vi "Set Velocity.vi"(0 "Process Variable(x)":dbl, 5 "Current TIme":u32, 7 "Current Power":dbl, 9 "Setpoint(end)":dbl, 11 "Total Distance":dbl format="%#_13g", 12 "Last Time Input":u32) -> (4 "Coerced Motor power":dbl format="%#_13g", 6 "End Loop?":bool=TRUE, 8 "Non-Coerced Motor Power":dbl, 10 "Last Time Output":u32)   [LabVIEW 2016]
panel:
  in  "Tick range":dbl=300.0 format="%#_13g"
  in  "Power Constant (power/ms^2) constant":dbl=0.0002 format="%#_13g"
  in  "Robot Barely Moving Power":dbl=0.3 format="%#_13g"
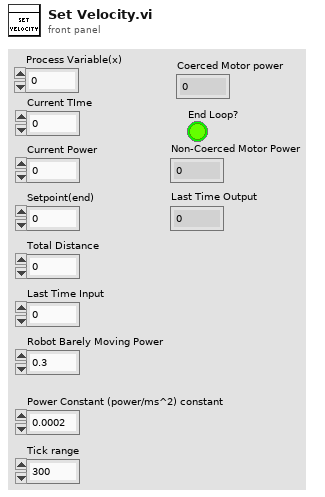
[diagram p1: front panel]
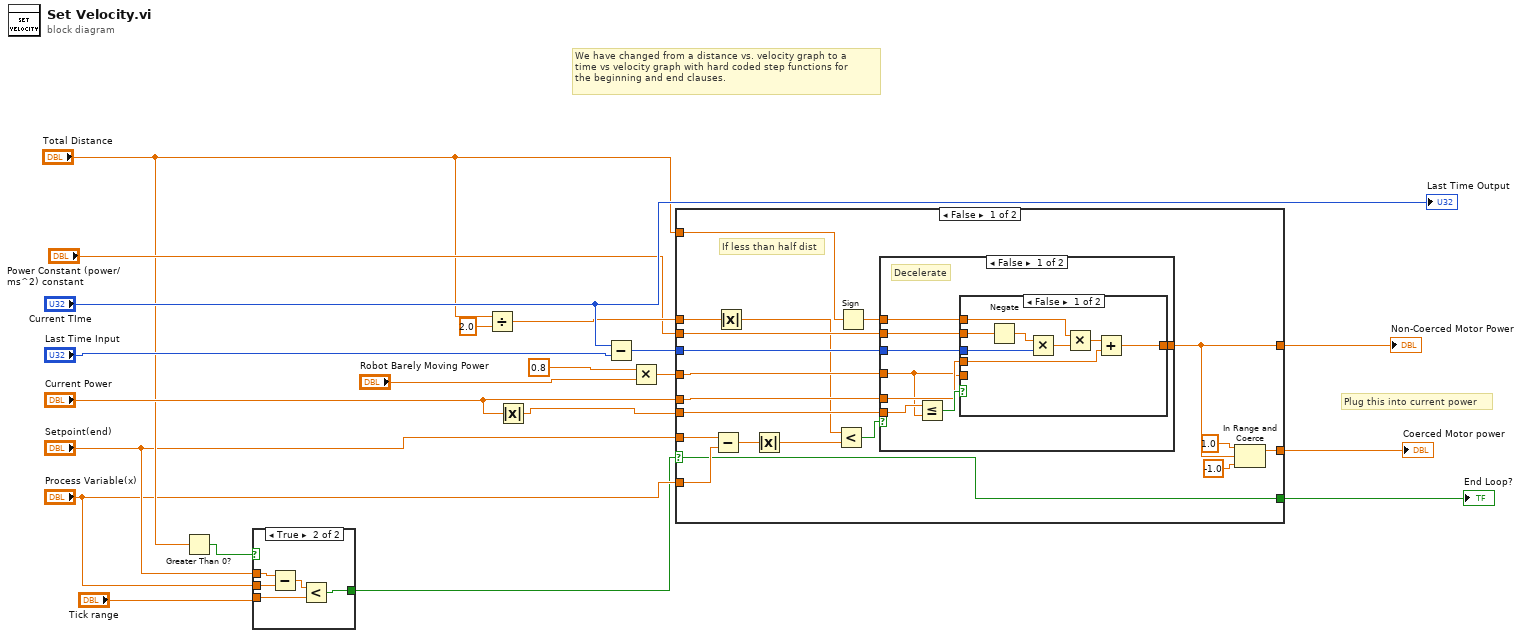
[diagram p0: block diagram]
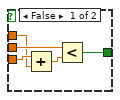
[diagram p2: hidden frame]
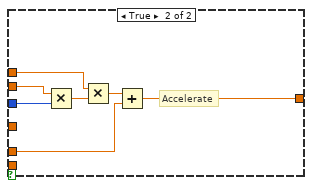
[diagram p4: hidden frame]
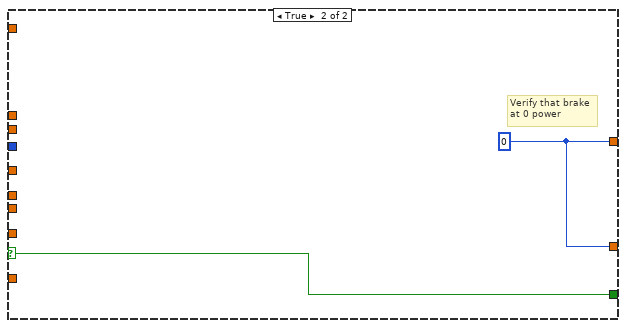
[diagram p5: hidden frame]
diagram:
  # "Plug this into current power"
  # "We have changed from a distance vs. velocity graph to a\ntime vs velocity graph with hard coded step functions for \nthe beginning and end clauses."
  n1 = Greater Than 0?(x="Total Distance") -> (x > 0?=w7:bool)
  n2 = case shown="True" w7 {
    tunnel: "Tick range" -> [w23 w30]
    tunnel: "Setpoint(end)" -> [w22 w29]
    tunnel: "Process Variable(x)" -> [w25 w28]
    tunnel: [w21 w26] -> w2
    frame False {
      n3 = Add(x=w23, y=w22) -> (x+y=w24:dbl)
      n4 = Less?(x=w25, y=w24) -> (x < y?=w21:bool)
    }
    frame True {
      n5 = Subtract(x=w29, y=w28) -> (x-y=w27:dbl)
      n6 = Less?(x=w27, y=w30) -> (x < y?=w26:bool)
    }
  }
  n7 = Divide(x="Total Distance", y=2.0) -> (x/y=w10:dbl)
  n8 = Absolute Value(x="Current Power") -> (abs(x)=w9:dbl)
  n9 = Subtract(x="Current TIme", y="Last Time Input") -> (x-y=w15:u32)
  n10 = Multiply(x=0.8, y="Robot Barely Moving Power") -> (x*y=w17:dbl)
  n11 = case shown="False" w2 {
    selector: w2 -> [w43 w75]
    tunnel: "Setpoint(end)" -> [w49 _]
    tunnel: "Process Variable(x)" -> [w48 _]
    tunnel: [w46 w74] -> w20
    tunnel: [w43 w75] -> w19
    tunnel: "Total Distance" -> [w41 _]
    tunnel: w10 -> [w40 _]
    tunnel: w17 -> [w36 _]
    tunnel: w15 -> [w39 _]
    tunnel: "Current Power" -> [w33 _]
    tunnel: w9 -> [w37 _]
    tunnel: "Power Constant (power/ms^2) constant" -> [w35 _]
    tunnel: [w32 w74] -> w1
    frame False {
      # "If less than half dist"
      n12 = Subtract(x=w49, y=w48) -> (x-y=w47:dbl)
      n13 = Absolute Value(x=w40) -> (abs(x)=w31:dbl)
      n14 = Absolute Value(x=w47) -> (abs(x)=w42:dbl)
      n15 = Less?(x=w31, y=w42) -> (x < y?=w38:bool)
      n16 = Sign(1:w41) -> (0:w34:dbl)
      n17 = case shown="False" w38 {
        tunnel: w39 -> [w53 w73]
        tunnel: [w55 w67] -> w32
        tunnel: w36 -> [w50 _]
        tunnel: w37 -> [w57 _]
        tunnel: w35 -> [w54 w71]
        tunnel: w34 -> [w52 w70]
        tunnel: w33 -> [w51 w68]
        frame False {
          # "Decelerate"
          n18 = Less Or Equal?(x=w57, y=w50) -> (x <= y?=w56:bool)
          n19 = case shown="False" w56 {
            tunnel: [w58 w66] -> w55
            tunnel: w50 -> [_ w66]
            tunnel: w54 -> [w64 _]
            tunnel: w53 -> [w63 _]
            tunnel: w52 -> [w61 _]
            tunnel: w51 -> [w59 _]
            frame False {
              n20 = Negate(x=w64) -> (-x=w65:dbl)
              n21 = Multiply(x=w65, y=w63) -> (x*y=w62:dbl)
              n22 = Multiply(x=w61, y=w62) -> (x*y=w60:dbl)
              n23 = Add(x=w60, y=w59) -> (x+y=w58:dbl)
            }
            frame True {
              # "Sets to barely moving power"
            }
          }
        }
        frame True {
          # "Accelerate"
          n24 = Multiply(x=w71, y=w73) -> (x*y=w72:dbl)
          n25 = Multiply(x=w70, y=w72) -> (x*y=w69:dbl)
          n26 = Add(x=w69, y=w68) -> (x+y=w67:dbl)
        }
      }
      n27 = In Range and Coerce(upper limit=1.0, x=w32, lower limit=-1.0) -> (coerced(x)=w46:dbl)  [unwired: 1 out]
    }
    frame True {
      w74 = 0
      # "Verify that brake\nat 0 power"
    }
  }
  "End Loop?" <- w19
  "Coerced Motor power" <- w20
  "Non-Coerced Motor Power" <- w1
  "Last Time Output" <- "Current TIme"
